vi "Test IDs.vi"() -> ()   [LabVIEW 2020]
uses:
  Address.ctl
  IDs.ctl
  Calibration Status.ctl
  Euler Angles.ctl
  Operating Mode.ctl
  <vilib>/MakerHub/LINX/Public/Utilities/Open Local.vi
  <vilib>/MakerHub/LINX/LMH-LINX.lvlib
  BNO055.lvclass
panel:
  out "Euler Angles":T1 {"Yaw" format="%.3f"; "Pitch" format="%.3f"; "Roll" format="%.3f"}
  out "Calibration":T2
  in  "Stop":bool
  out "Device Name":string
  in  "I2C Bus":u8=1
  out "IDs":T3 {"Gyro ID" format="0x%02x"; "Mag ID" format="0x%02x"; "Acc ID" format="0x%02x"; "Chip ID" format="0x%02x"}
  in  "IMU Addr":T4=40 items=["0x28"=40, "0x29"=41]
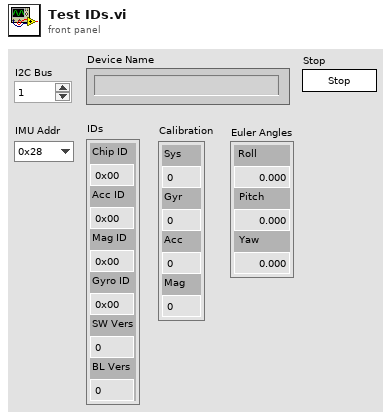
[diagram p1: front panel]
types:
  T1 = typedef "BNO055.lvlib/BNO055.lvclass/Euler Angles.ctl" = cluster{"Roll":dbl, "Pitch":dbl, "Yaw":dbl}
  T2 = typedef "BNO055.lvlib/BNO055.lvclass/Calibration Status.ctl" = cluster{"Sys":u8, "Gyr":u8, "Acc":u8, "Mag":u8}
  T3 = typedef "BNO055.lvlib/BNO055.lvclass/IDs.ctl" = cluster{"Chip ID":u8, "Acc ID":u8, "Mag ID":u8, "Gyro ID":u8, "SW Vers":u16, "BL Vers":u8}
  T4 = typedef "BNO055.lvlib/BNO055.lvclass/Address.ctl" = u8
  T5 = typedef "LMH-LINX.lvlib/LINX Ref.ctl" = cluster{"IO":T6, "Interface":T7, "LINX Device Config":T8}
  T6 = typedef "LMH-LINX.lvlib/Platform.ctl" = enum16{"Remote", "Local"}
  T7 = typedef "LMH-LINX.lvlib/Interface.ctl" = enum16{"Serial", "TCP"}
  T8 = typedef "LMH-LINX.lvlib/Device.lvlib/LINX Device Config.ctl" = cluster{"Interface":T7, "COM Port":refnum<visa-resource-name>, "TCP Configuration":T9, "Device Family":u8, "Device ID":u8, "Device Name":string, "TCP Ref":refnum<k5>, "Channels":T10}
  T9 = typedef "LMH-LINX.lvlib/Device.lvlib/TCP Config.ctl" = cluster{"IP Address":string, "Port":u16}
  T10 = typedef "LMH-LINX.lvlib/Channels.ctl" = cluster{"DI":u8[], "DO":u8[], "AI":u8[], "AO":u8[], "PWM":u8[], "QE":u8[], "UART":u8[], "I2C 2":u8[], "SPI":u8[], "CAN":u8[], "Servo":u8[], "AI Ref (V)":dbl, "AI Resolution (Bits)":u8, "AO Ref (V)":dbl, "AO Resolution (Bits)":u8}
  T11 = typedef "BNO055.lvlib/BNO055.lvclass/Operating Mode.ctl" = enum8{"Config", "Acc Only", "Mag Only", "Gyr Only", "Acc Mag", "Acc Gyr", "Mag Gyr", "AccMagGyr", "IMU", "Compass", "Mag4Gyr", "NDOF FMC Off", "NDOF"}
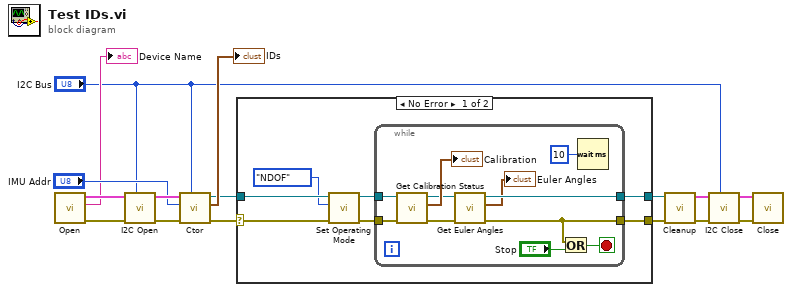
[diagram p0: block diagram]
diagram:
  n1 = call-poly <vilib>:"Open.vi"() -> ("Error Out"=w15:errorcluster, "Device Name"=→"Device Name":string, "LINX Resource"=w16:T5)  [unwired: 9 in]
  n2 = call <vilib>:"I2C Open.vi"("I2C Channel (0)"="I2C Bus", "Error In"=w15, "LINX Resource"=w16) -> ("Error Out"=w13:errorcluster, "LINX Resource"=w14:T5)  [unwired: 7 in]
  n3 = call "Ctor.vi"("I2C Channel"="I2C Bus", "error in (no error)"=w13, "Address"="IMU Addr", "LINX Resource"=w14) -> ("error out"=w4:errorcluster, "IDs"=→"IDs":T3, "BNO055 out"=w3:refnum<class "BNO055.lvclass">)  [unwired: 5 in]
  n4 = case shown="No Error" w4 {
    selector: w4 -> [w22 w35]
    tunnel: w3 -> [w23 w36]
    tunnel: [w17 w36] -> w2
    tunnel: [w18 w35] -> w1
    frame No Error {
      n5 = call "Set Operating Mode.vi"("error in (no error)"=w22, "Operating Mode"=Operating_Mode."NDOF", "BNO055 in"=w23) -> ("error out"=w19:errorcluster, "BNO055 out"=w20:refnum<class "BNO055.lvclass">)  [unwired: 7 in]
      n6 = while {
        tunnel: w19 -> [w30]
        tunnel: w20 -> [w31]
        tunnel: [w25] -> w18
        tunnel: [w26] -> w17
        stop <- w33 stop-if-true
        n7 = call "Get Calibration Status.vi"("error in (no error)"=w30, "BNO055 in"=w31) -> ("error out"=w27:errorcluster, "Calibration Status"=→"Calibration":T2, "BNO055 out"=w28:refnum<class "BNO055.lvclass">)  [unwired: 7 in]
        n8 = call "Get Euler Angles.vi"("error in (no error)"=w27, "BNO055 in"=w28) -> ("error out"=w25:errorcluster, "Euler Angles"=→"Euler Angles":T1, "BNO055 out"=w26:refnum<class "BNO055.lvclass">)  [unwired: 7 in]
        n9 = Or(x=w25, y="Stop") -> (x .or. y?=w33:bool)
        n10 = Wait (ms)(milliseconds to wait=u32 10) -> ()  [unwired: 1 out]
      }
    }
    frame Error {
    }
  }
  n11 = call "Cleanup.vi"("error in (no error)"=w1, "BNO055 in"=w2) -> ("error out"=w9:errorcluster, "LINX Resource"=w10:T5)  [unwired: 8 in]
  n12 = call <vilib>:"I2C Close.vi"("I2C Channel (0)"="I2C Bus", "Error In"=w9, "LINX Resource"=w10) -> ("Error Out"=w7:errorcluster, "LINX Resource"=w8:T5)  [unwired: 7 in]
  n13 = call <vilib>:"Close.vi"("Error In"=w7, "LINX Resource"=w8) -> ()  [unwired: 9 in, 1 out]
